vi "VOC.vi"(0 "input VOC ports":u8[](array[numeric]), 1 "voc states array":cluster{u32, u8}[](array[cluster]), 5 "output VOC ports":u8[](array[numeric]), 7 "Input VOC msg Array":T1(array[cluster]), 9 "output VOC msg array":T1(array[cluster])) -> (3 "Filled voc states array":cluster{u32, u8}[](array[cluster]), 4 "Modified input VOC ports":u8[](array[numeric]), 6 "Modified output VOC ports":u8[](array[numeric]), 8 "Clear Input VOC msg Array":T1(array[cluster]), 10 "output VOC array":T1(array[cluster]))   [LabVIEW 2010]
uses:
  New debug prog (1)/New debug prog/VOC/voc.dll
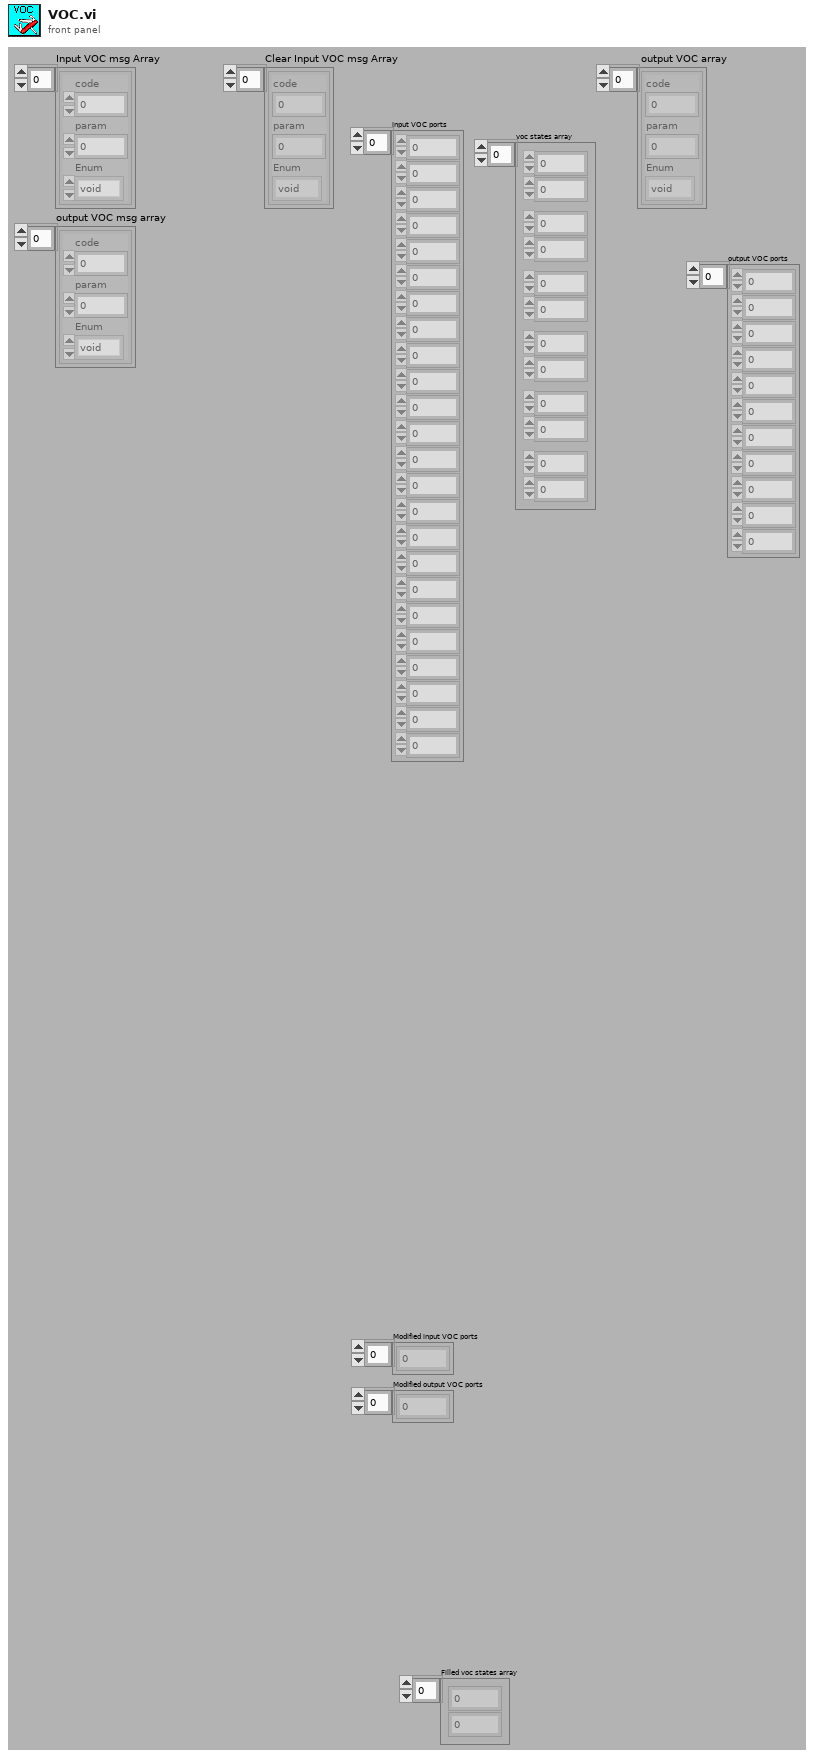
[diagram p1: front panel]
types:
  T1 = cluster{"code":i32, "param":i32, "Enum":enum16{"void", "byte", "int", "float"}}[]
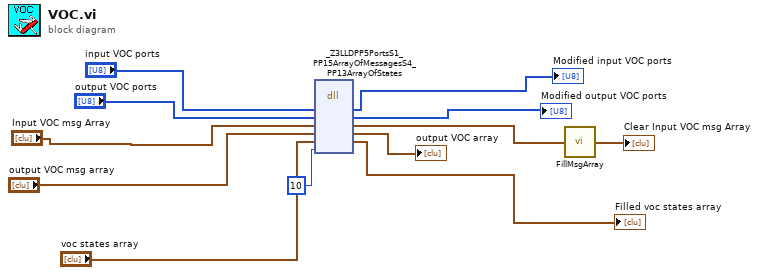
[diagram p0: block diagram]
diagram:
  n1 = dll-call lib="D:/Liakh Tanya/Dissertation/Complex/Old debug progs/New debug prog (1)/New debug prog/VOC/voc.dll" fn="_Z3LLDPP5PortsS1_PP15ArrayOfMessagesS4_PP13ArrayOfStates" label="VOC"("input"="input VOC ports", "output"="output VOC ports", "msg_inp"="Input VOC msg Array", "msg_inp"="output VOC msg array", "arg5"="voc states array", "steps"=u32 10) -> ("input"=→"Modified input VOC ports":i8[], "output"=→"Modified output VOC ports":i8[], "msg_inp"=w2:T1, "msg_inp"=→"output VOC array":T1, "arg5"=→"Filled voc states array":cluster{u32, u8}[])  [unwired: 5 in, 2 out]
  n2 = call "FillMsgArray.vi"("Input VOC msg Array"=w2) -> ("Clear msg Array"=→"Clear Input VOC msg Array":T1)
